vi "LoadConfig.vi"(11 "configuration file":path) -> ()   [LabVIEW 2012]
uses:
  <vilib>/Utility/config.llb/Read Key (Path).vi
  variables/GlobalUI.vi
  <vilib>/Utility/config.llb/Read Key (U32).vi
  <vilib>/Utility/config.llb/Read Key (Double).vi
  <vilib>/Utility/config.llb/Read Key (I32).vi
  <vilib>/Utility/config.llb/Read Key (String).vi
  <vilib>/Utility/config.llb/NI_LVConfig.lvlib
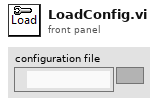
[diagram p1: front panel]
types:
  T1 = typedef "NI_LVConfig.lvlib/Config Data RefNum.ctl" = refnum<k1>
  T2 = typedef "Scan Parameters.ctl" = cluster{"x pixels":i32, "x voltage min":dbl, "x voltage max":dbl, "y voltage min":dbl, "y voltage max":dbl, "fill frac":dbl, "Zoom":dbl, "BiDi":bool, "scan rate (ms/line)":dbl}
  T3 = typedef "HWsettings.ctl" = cluster{"Galvo Channels":tag, "Detector Channels":tag, "Galvo Trigger":tag, "Shutter Lines":tag[], "Max Acquisition Rate":dbl, "Recommended Acquisition Rate":dbl, "Galvo Write Rate":dbl, "Max Timebase Frequency (Hz)":dbl, "MCC Shutter Lines":refnum<k21>[], "Detector Task":refnum<k21>, "Shutter Tasks":refnum<k21>[], "Galvo Task":refnum<k21>, "Digital Image Multiplier":dbl[]}
  T4 = typedef "Stage Parameters.ctl" = cluster{"Scan Mode":T5, "Start position mm":dbl, "End position mm":dbl, "Velocity um/sec (continuous)":dbl, "Step size microns (discrete)":dbl, "Frames to grab (grab)":i32}
  T5 = typedef "ScanMode.ctl" = enum16{"None", "Continuous", "Point Scan (CH3 cursor)", "Point Scan Move (CH3 cursor)", "Grab", "Grab Move Stage", "Grab Move Z-stage", "Cont. Move Z-stage", "Spec Move Stage", "Spec Move Cont", "Surf Calib"}
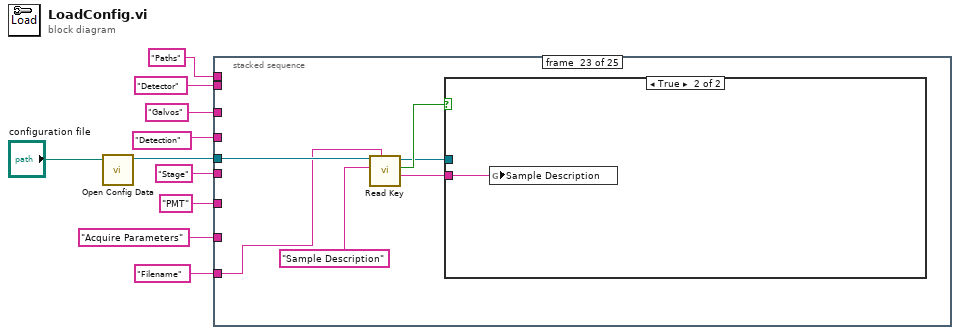
[diagram p0: block diagram]
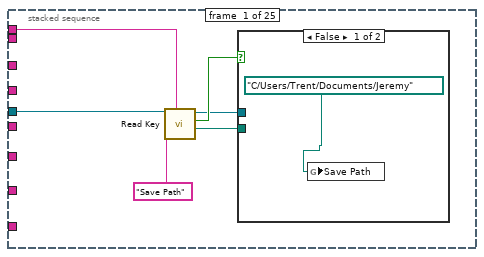
[diagram p2: hidden frame]
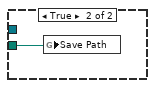
[diagram p3: hidden frame]
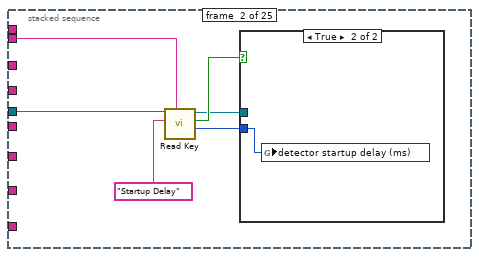
[diagram p4: hidden frame]
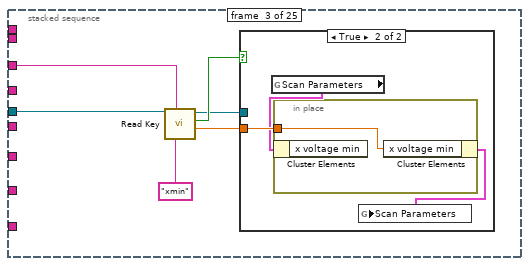
[diagram p6: hidden frame]
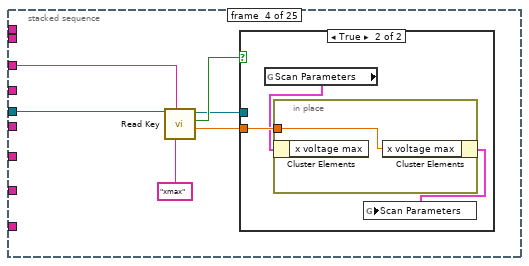
[diagram p8: hidden frame]
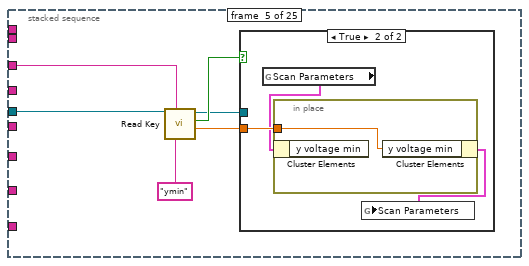
[diagram p10: hidden frame]
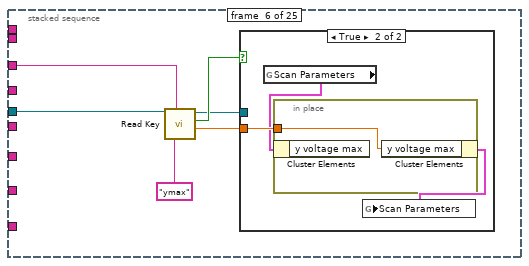
[diagram p12: hidden frame]
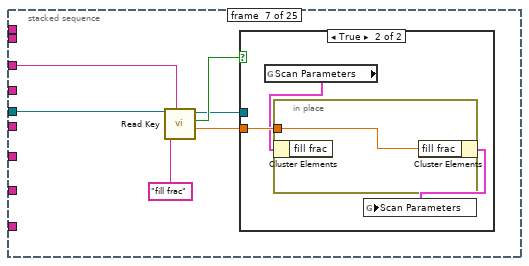
[diagram p14: hidden frame]
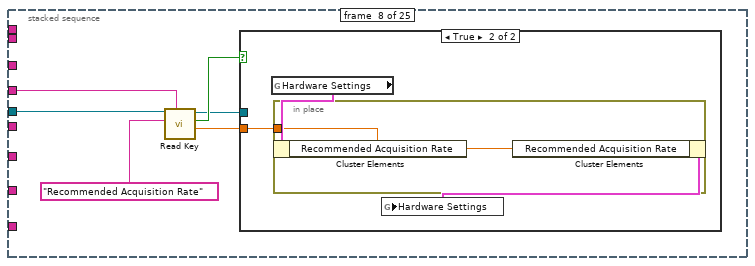
[diagram p16: hidden frame]
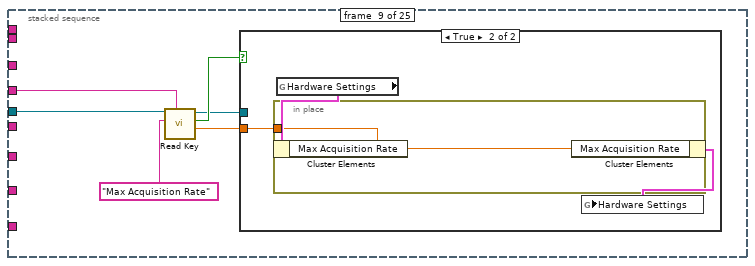
[diagram p18: hidden frame]
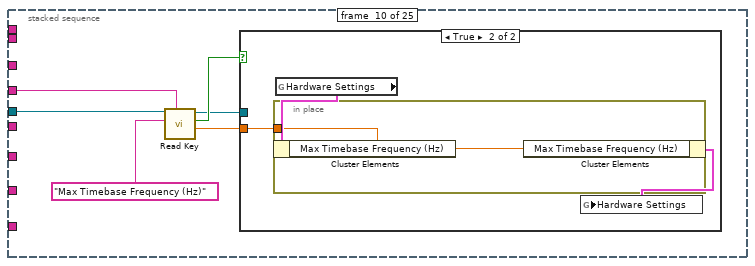
[diagram p20: hidden frame]
diagram:
  n1 = call <vilib>:"Open Config Data.vi"("configuration file path"="configuration file") -> ("refnum"=w10:T1)  [unwired: 8 in, 2 out]
  n2 = stacked-sequence {
    tunnel: w10 -> [w16 w24 w31 w41 w51 w61 w71 w81 w91 w101 w111 w118 w125 w132 w139 w146 w153 w160 w170 w180 w190 w200 w210 w217 w224]
    tunnel: "Detection" ("section") -> [_ _ _ _ _ _ _ w76 w86 w96 _ _ _ _ _ _ _ _ _ _ _ _ _ _ _]
    tunnel: "Galvos" ("section") -> [_ _ w26 w36 w46 w56 w66 _ _ _ _ _ _ _ _ _ _ _ _ _ _ _ _ _ _]
    tunnel: "Detector" ("section") -> [_ w19 _ _ _ _ _ _ _ _ _ _ _ _ _ _ _ _ _ _ _ _ _ _ _]
    tunnel: "Paths" ("section") -> [w11 _ _ _ _ _ _ _ _ _ _ _ _ _ _ _ _ _ _ _ _ _ _ _ _]
    tunnel: "Stage" ("section") -> [_ _ _ _ _ _ _ _ _ _ w106 w113 w120 w127 _ _ _ _ _ _ _ _ _ _ _]
    tunnel: "PMT" ("section") -> [_ _ _ _ _ _ _ _ _ _ _ _ _ _ w134 w141 w148 _ _ _ _ _ _ _ _]
    tunnel: "Acquire Parameters" ("section") -> [_ _ _ _ _ _ _ _ _ _ _ _ _ _ _ _ _ w155 w165 w175 w185 w195 _ _ _]
    tunnel: "Filename" ("section") -> [_ _ _ _ _ _ _ _ _ _ _ _ _ _ _ _ _ _ _ _ _ _ w205 w212 w219]
    frame #0 {
      n3 = call-poly <vilib>:"Read Key.vi"("section"=w11, "key"="Save Path", "refnum"=w16) -> ("value"=w13:path, "found?"=w14:bool, "refnum out"=w12:T1)  [unwired: 5 in, 1 out]
      n4 = case shown="False" w14 {
        tunnel: w13 -> [_ w18]
        tunnel: w12 -> [_ _]
        frame False {
          n5 = global write "GlobalUI.vi" "Save Path"(path "C:/Users/Trent/Documents/Jeremy" ("Save Path")) -> ()
        }
        frame True {
          n6 = global write "GlobalUI.vi" "Save Path"(w18) -> ()
        }
      }
    }
    frame #1 {
      n7 = call-poly <vilib>:"Read Key.vi"("section"=w19, "key"="Startup Delay", "refnum"=w24) -> ("value"=w21:u32, "found?"=w22:bool, "refnum out"=w20:T1)  [unwired: 5 in, 1 out]
      n8 = case shown="True" w22 {
        tunnel: w21 -> [_ w25]
        tunnel: w20 -> [_ _]
        frame False {
        }
        frame True {
          n9 = global write "GlobalUI.vi" "detector startup delay (ms)"(w25) -> ()
        }
      }
    }
    frame #2 {
      n10 = call-poly <vilib>:"Read Key.vi"("section"=w26, "key"="xmin", "refnum"=w31) -> ("value"=w28:dbl, "found?"=w29:bool, "refnum out"=w27:T1)  [unwired: 5 in, 1 out]
      n11 = case shown="True" w29 {
        tunnel: w28 -> [_ w34]
        tunnel: w27 -> [_ _]
        frame False {
        }
        frame True {
          n12 = global read "GlobalUI.vi" "Scan Parameters"() -> (w32:T2)
          n13 = in-place {
            in-place-border: w34 -> [w35]
            n14 = in-place-cluster #1(w32) -> ()  [unwired: 1 out]
            n15 = in-place-cluster #1("x voltage min"=w35) -> (w33:T2)
          }
          n16 = global write "GlobalUI.vi" "Scan Parameters"(w33) -> ()
        }
      }
    }
    frame #3 {
      n17 = call-poly <vilib>:"Read Key.vi"("section"=w36, "key"="xmax", "refnum"=w41) -> ("value"=w38:dbl, "found?"=w39:bool, "refnum out"=w37:T1)  [unwired: 5 in, 1 out]
      n18 = case shown="True" w39 {
        tunnel: w38 -> [_ w44]
        tunnel: w37 -> [_ _]
        frame False {
        }
        frame True {
          n19 = global read "GlobalUI.vi" "Scan Parameters"() -> (w43:T2)
          n20 = in-place {
            in-place-border: w44 -> [w45]
            n21 = in-place-cluster #2(w43) -> ()  [unwired: 1 out]
            n22 = in-place-cluster #2("x voltage max"=w45) -> (w42:T2)
          }
          n23 = global write "GlobalUI.vi" "Scan Parameters"(w42) -> ()
        }
      }
    }
    frame #4 {
      n24 = call-poly <vilib>:"Read Key.vi"("section"=w46, "key"="ymin", "refnum"=w51) -> ("value"=w48:dbl, "found?"=w49:bool, "refnum out"=w47:T1)  [unwired: 5 in, 1 out]
      n25 = case shown="True" w49 {
        tunnel: w48 -> [_ w54]
        tunnel: w47 -> [_ _]
        frame False {
        }
        frame True {
          n26 = global read "GlobalUI.vi" "Scan Parameters"() -> (w53:T2)
          n27 = in-place {
            in-place-border: w54 -> [w55]
            n28 = in-place-cluster #3(w53) -> ()  [unwired: 1 out]
            n29 = in-place-cluster #3("y voltage min"=w55) -> (w52:T2)
          }
          n30 = global write "GlobalUI.vi" "Scan Parameters"(w52) -> ()
        }
      }
    }
    frame #5 {
      n31 = call-poly <vilib>:"Read Key.vi"("section"=w56, "key"="ymax", "refnum"=w61) -> ("value"=w58:dbl, "found?"=w59:bool, "refnum out"=w57:T1)  [unwired: 5 in, 1 out]
      n32 = case shown="True" w59 {
        tunnel: w58 -> [_ w64]
        tunnel: w57 -> [_ _]
        frame False {
        }
        frame True {
          n33 = global read "GlobalUI.vi" "Scan Parameters"() -> (w63:T2)
          n34 = in-place {
            in-place-border: w64 -> [w65]
            n35 = in-place-cluster #4(w63) -> ()  [unwired: 1 out]
            n36 = in-place-cluster #4("y voltage max"=w65) -> (w62:T2)
          }
          n37 = global write "GlobalUI.vi" "Scan Parameters"(w62) -> ()
        }
      }
    }
    frame #6 {
      n38 = call-poly <vilib>:"Read Key.vi"("section"=w66, "key"="fill frac", "refnum"=w71) -> ("value"=w68:dbl, "found?"=w69:bool, "refnum out"=w67:T1)  [unwired: 5 in, 1 out]
      n39 = case shown="True" w69 {
        tunnel: w68 -> [_ w74]
        tunnel: w67 -> [_ _]
        frame False {
        }
        frame True {
          n40 = global read "GlobalUI.vi" "Scan Parameters"() -> (w73:T2)
          n41 = in-place {
            in-place-border: w74 -> [w75]
            n42 = in-place-cluster #5(w73) -> ()  [unwired: 1 out]
            n43 = in-place-cluster #5("fill frac"=w75) -> (w72:T2)
          }
          n44 = global write "GlobalUI.vi" "Scan Parameters"(w72) -> ()
        }
      }
    }
    frame #7 {
      n45 = call-poly <vilib>:"Read Key.vi"("section"=w76, "key"="Recommended Acquisition Rate", "refnum"=w81) -> ("value"=w78:dbl, "found?"=w79:bool, "refnum out"=w77:T1)  [unwired: 5 in, 1 out]
      n46 = case shown="True" w79 {
        tunnel: w78 -> [_ w84]
        tunnel: w77 -> [_ _]
        frame False {
        }
        frame True {
          n47 = global read "GlobalUI.vi" "Hardware Settings"() -> (w83:T3)
          n48 = in-place {
            in-place-border: w84 -> [w85]
            n49 = in-place-cluster #6(w83) -> ()  [unwired: 1 out]
            n50 = in-place-cluster #6("Recommended Acquisition Rate"=w85) -> (w82:T3)
          }
          n51 = global write "GlobalUI.vi" "Hardware Settings"(w82) -> ()
        }
      }
    }
    frame #8 {
      n52 = call-poly <vilib>:"Read Key.vi"("section"=w86, "key"="Max Acquisition Rate", "refnum"=w91) -> ("value"=w88:dbl, "found?"=w89:bool, "refnum out"=w87:T1)  [unwired: 5 in, 1 out]
      n53 = case shown="True" w89 {
        tunnel: w88 -> [_ w94]
        tunnel: w87 -> [_ _]
        frame False {
        }
        frame True {
          n54 = global read "GlobalUI.vi" "Hardware Settings"() -> (w93:T3)
          n55 = in-place {
            in-place-border: w94 -> [w95]
            n56 = in-place-cluster #7(w93) -> ()  [unwired: 1 out]
            n57 = in-place-cluster #7("Max Acquisition Rate"=w95) -> (w92:T3)
          }
          n58 = global write "GlobalUI.vi" "Hardware Settings"(w92) -> ()
        }
      }
    }
    frame #9 {
      n59 = call-poly <vilib>:"Read Key.vi"("section"=w96, "key"="Max Timebase Frequency (Hz)", "refnum"=w101) -> ("value"=w98:dbl, "found?"=w99:bool, "refnum out"=w97:T1)  [unwired: 5 in, 1 out]
      n60 = case shown="True" w99 {
        tunnel: w98 -> [_ w104]
        tunnel: w97 -> [_ _]
        frame False {
        }
        frame True {
          n61 = global read "GlobalUI.vi" "Hardware Settings"() -> (w102:T3)
          n62 = in-place {
            in-place-border: w104 -> [w105]
            n63 = in-place-cluster #8(w102) -> ()  [unwired: 1 out]
            n64 = in-place-cluster #8("Max Timebase Frequency (Hz)"=w105) -> (w103:T3)
          }
          n65 = global write "GlobalUI.vi" "Hardware Settings"(w103) -> ()
        }
      }
    }
    frame #10 {
      n66 = call-poly <vilib>:"Read Key.vi"("section"=w106, "key"="Serial Number", "refnum"=w111) -> ("value"=w108:i32, "found?"=w109:bool, "refnum out"=w107:T1)  [unwired: 5 in, 1 out]
      n67 = case shown="True" w109 {
        tunnel: w108 -> [_ w112]
        tunnel: w107 -> [_ _]
        frame False {
        }
        frame True {
          n68 = global write "GlobalUI.vi" "Stage Serial Number"(w112) -> ()
        }
      }
    }
    frame #11 {
      n69 = call-poly <vilib>:"Read Key.vi"("section"=w113, "key"="Target1", "refnum"=w118) -> ("value"=w115:dbl, "found?"=w116:bool, "refnum out"=w114:T1)  [unwired: 5 in, 1 out]
      n70 = case shown="True" w116 {
        tunnel: w115 -> [_ w119]
        tunnel: w114 -> [_ _]
        frame False {
        }
        frame True {
          n71 = global write "GlobalUI.vi" "Target position mm"(w119) -> ()
        }
      }
    }
    frame #12 {
      n72 = call-poly <vilib>:"Read Key.vi"("section"=w120, "key"="Target2", "refnum"=w125) -> ("value"=w122:dbl, "found?"=w123:bool, "refnum out"=w121:T1)  [unwired: 5 in, 1 out]
      n73 = case shown="True" w123 {
        tunnel: w122 -> [_ w126]
        tunnel: w121 -> [_ _]
        frame False {
        }
        frame True {
          n74 = global write "GlobalUI.vi" "Target position mm 2"(w126) -> ()
        }
      }
    }
    frame #13 {
      n75 = call-poly <vilib>:"Read Key.vi"("section"=w127, "key"="Target3", "refnum"=w132) -> ("value"=w129:dbl, "found?"=w130:bool, "refnum out"=w128:T1)  [unwired: 5 in, 1 out]
      n76 = case shown="True" w130 {
        tunnel: w129 -> [_ w133]
        tunnel: w128 -> [_ _]
        frame False {
        }
        frame True {
          n77 = global write "GlobalUI.vi" "Target position mm 3"(w133) -> ()
        }
      }
    }
    frame #14 {
      n78 = call-poly <vilib>:"Read Key.vi"("section"=w134, "key"="V1", "refnum"=w139) -> ("value"=w136:dbl, "found?"=w137:bool, "refnum out"=w135:T1)  [unwired: 5 in, 1 out]
      n79 = case shown="True" w137 {
        tunnel: w136 -> [_ w140]
        tunnel: w135 -> [_ _]
        frame False {
        }
        frame True {
          n80 = global write "GlobalUI.vi" "PMT1"(w140) -> ()
        }
      }
    }
    frame #15 {
      n81 = call-poly <vilib>:"Read Key.vi"("section"=w141, "key"="V2", "refnum"=w146) -> ("value"=w143:dbl, "found?"=w144:bool, "refnum out"=w142:T1)  [unwired: 5 in, 1 out]
      n82 = case shown="True" w144 {
        tunnel: w143 -> [_ w147]
        tunnel: w142 -> [_ _]
        frame False {
        }
        frame True {
          n83 = global write "GlobalUI.vi" "PMT2"(w147) -> ()
        }
      }
    }
    frame #16 {
      n84 = call-poly <vilib>:"Read Key.vi"("section"=w148, "key"="V3", "refnum"=w153) -> ("value"=w150:dbl, "found?"=w151:bool, "refnum out"=w149:T1)  [unwired: 5 in, 1 out]
      n85 = case shown="True" w151 {
        tunnel: w150 -> [_ w154]
        tunnel: w149 -> [_ _]
        frame False {
        }
        frame True {
          n86 = global write "GlobalUI.vi" "PMT3"(w154) -> ()
        }
      }
    }
    frame #17 {
      n87 = call-poly <vilib>:"Read Key.vi"("section"=w155, "key"="Start", "refnum"=w160) -> ("value"=w157:dbl, "found?"=w158:bool, "refnum out"=w156:T1)  [unwired: 5 in, 1 out]
      n88 = case shown="True" w158 {
        tunnel: w157 -> [_ w162]
        tunnel: w156 -> [_ _]
        frame False {
        }
        frame True {
          n89 = global read "GlobalUI.vi" "Stage Acquire Parameters"() -> (w163:T4)
          n90 = in-place {
            in-place-border: w162 -> [w164]
            n91 = in-place-cluster #9(w163) -> ()  [unwired: 1 out]
            n92 = in-place-cluster #9("Start position mm"=w164) -> (w161:T4)
          }
          n93 = global write "GlobalUI.vi" "Stage Acquire Parameters"(w161) -> ()
        }
      }
    }
    frame #18 {
      n94 = call-poly <vilib>:"Read Key.vi"("section"=w165, "key"="End", "refnum"=w170) -> ("value"=w167:dbl, "found?"=w168:bool, "refnum out"=w166:T1)  [unwired: 5 in, 1 out]
      n95 = case shown="True" w168 {
        tunnel: w167 -> [_ w172]
        tunnel: w166 -> [_ _]
        frame False {
        }
        frame True {
          n96 = global read "GlobalUI.vi" "Stage Acquire Parameters"() -> (w173:T4)
          n97 = in-place {
            in-place-border: w172 -> [w174]
            n98 = in-place-cluster #10(w173) -> ()  [unwired: 1 out]
            n99 = in-place-cluster #10("End position mm"=w174) -> (w171:T4)
          }
          n100 = global write "GlobalUI.vi" "Stage Acquire Parameters"(w171) -> ()
        }
      }
    }
    frame #19 {
      n101 = call-poly <vilib>:"Read Key.vi"("section"=w175, "key"="Velocity", "refnum"=w180) -> ("value"=w177:dbl, "found?"=w178:bool, "refnum out"=w176:T1)  [unwired: 5 in, 1 out]
      n102 = case shown="True" w178 {
        tunnel: w177 -> [_ w182]
        tunnel: w176 -> [_ _]
        frame False {
        }
        frame True {
          n103 = global read "GlobalUI.vi" "Stage Acquire Parameters"() -> (w183:T4)
          n104 = in-place {
            in-place-border: w182 -> [w184]
            n105 = in-place-cluster #11(w183) -> ()  [unwired: 1 out]
            n106 = in-place-cluster #11("Velocity um/sec (continuous)"=w184) -> (w181:T4)
          }
          n107 = global write "GlobalUI.vi" "Stage Acquire Parameters"(w181) -> ()
        }
      }
    }
    frame #20 {
      n108 = call-poly <vilib>:"Read Key.vi"("section"=w185, "key"="Step size", "refnum"=w190) -> ("value"=w187:dbl, "found?"=w188:bool, "refnum out"=w186:T1)  [unwired: 5 in, 1 out]
      n109 = case shown="True" w188 {
        tunnel: w187 -> [_ w192]
        tunnel: w186 -> [_ _]
        frame False {
        }
        frame True {
          n110 = global read "GlobalUI.vi" "Stage Acquire Parameters"() -> (w193:T4)
          n111 = in-place {
            in-place-border: w192 -> [w194]
            n112 = in-place-cluster #12(w193) -> ()  [unwired: 1 out]
            n113 = in-place-cluster #12("Step size microns (discrete)"=w194) -> (w191:T4)
          }
          n114 = global write "GlobalUI.vi" "Stage Acquire Parameters"(w191) -> ()
        }
      }
    }
    frame #21 {
      n115 = call-poly <vilib>:"Read Key.vi"("section"=w195, "key"="Frames to grab", "refnum"=w200) -> ("value"=w197:i32, "found?"=w198:bool, "refnum out"=w196:T1)  [unwired: 5 in, 1 out]
      n116 = case shown="True" w198 {
        tunnel: w197 -> [_ w202]
        tunnel: w196 -> [_ _]
        frame False {
        }
        frame True {
          n117 = global read "GlobalUI.vi" "Stage Acquire Parameters"() -> (w203:T4)
          n118 = in-place {
            in-place-border: w202 -> [w204]
            n119 = in-place-cluster #13(w203) -> ()  [unwired: 1 out]
            n120 = in-place-cluster #13("Frames to grab (grab)"=w204) -> (w201:T4)
          }
          n121 = global write "GlobalUI.vi" "Stage Acquire Parameters"(w201) -> ()
        }
      }
    }
    frame #22 {
      n122 = call-poly <vilib>:"Read Key.vi"("section"=w205, "key"="Sample Description", "refnum"=w210) -> ("value"=w207:string, "found?"=w208:bool, "refnum out"=w206:T1)  [unwired: 5 in, 1 out]
      n123 = case shown="True" w208 {
        tunnel: w207 -> [_ w211]
        tunnel: w206 -> [_ _]
        frame False {
        }
        frame True {
          n124 = global write "GlobalUI.vi" "Sample Description"(w211) -> ()
        }
      }
    }
    frame #23 {
      n125 = call-poly <vilib>:"Read Key.vi"("section"=w212, "key"="Pump Power", "refnum"=w217) -> ("value"=w214:string, "found?"=w215:bool, "refnum out"=w213:T1)  [unwired: 5 in, 1 out]
      n126 = case shown="True" w215 {
        tunnel: w214 -> [_ w218]
        tunnel: w213 -> [_ _]
        frame False {
        }
        frame True {
          n127 = global write "GlobalUI.vi" "Pump Power (mW)"(w218) -> ()
        }
      }
    }
    frame #24 {
      n128 = call-poly <vilib>:"Read Key.vi"("section"=w219, "key"="Stokes Power", "refnum"=w224) -> ("value"=w221:string, "found?"=w222:bool, "refnum out"=w220:T1)  [unwired: 5 in, 1 out]
      n129 = case shown="True" w222 {
        tunnel: w221 -> [_ w225]
        tunnel: w220 -> [_ _]
        frame False {
        }
        frame True {
          n130 = global write "GlobalUI.vi" "Stokes Power (mW)"(w225) -> ()
        }
      }
    }
  }
